vi "Create All Message Queues.vi"(8 "error in (no error)":T1 caption="entrée d'erreur (pas d'erreur)") -> (0 "error out":T1 caption="sortie d'erreur", 3 "Files d'attente de messages en sortie":T2)   [LabVIEW 2020, in "Message Queue.lvlib"]
doc: "Ce VI crée et initialise toutes les files d'attente de messages de l'application. Si votre application requiert plusieurs files d'attente de messages, cliquez sur la constante \"Message Queues\" ci-dessus avec le bouton droit et sélectionnez Ouvrir la déf. de type. Ajoutez les nouvelles files d'attente de messages à la définition de type puis initialisez-les dans ce VI."
uses:
  Message Queue.lvlib
  All Message Queues.ctl
  Message Cluster.ctl
  Enqueue Message (Single).vi
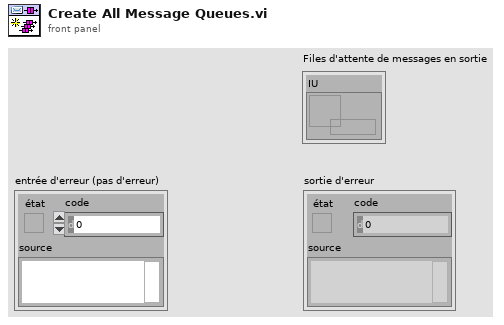
[diagram p1: front panel]
types:
  T1 = cluster{"état":bool, "code":i32, "source":string}
  T2 = typedef "Message Queue.lvlib/All Message Queues.ctl" = cluster{"IU":refnum<queue>}
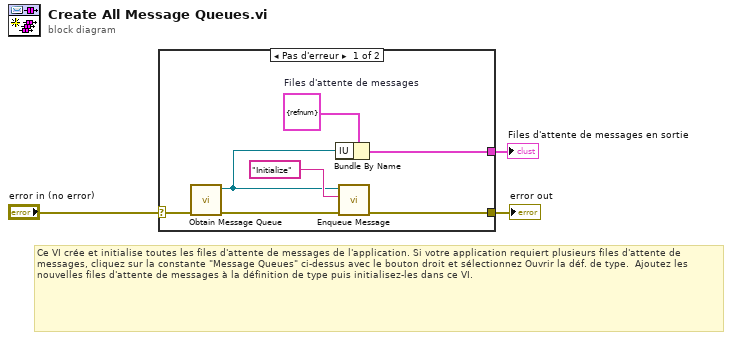
[diagram p0: block diagram]
diagram:
  # "Ce VI crée et initialise toutes les files d'attente de messages de l'application. Si votre application requiert plusieurs files d'attente de messages, cliquez sur la constante \"Message Queues\" ci-dessus avec le bouton droit et sélectionnez Ouvrir la déf. de type.  Ajoutez les nouvelles files d'attente de messages à la définition de type puis initialisez-les dans ce VI."
  n1 = case shown="Pas d'erreur" "error in (no error)" {
    selector: "error in (no error)" -> [w7 w11]
    tunnel: [w10 w11] -> w3
    tunnel: [w8 _] -> w2
    frame No Error {
      w9 = T2 {"IU"=refnum}  # Files d'attente de messages
      n2 = call "Obtain Message Queue.vi"("error in (no error)"=w7) -> ("error out"=w6:T1, "File d'attente de messages"=w4:refnum<queue>)  [unwired: 9 in]
      n3 = Bundle By Name(cluster=w9, "IU"=w4) -> (w8:T2)
      n4 = call-poly "Enqueue Message.vi"("error in (no error)"=w6, "Message"="Initialize", "File d'attente de messages"=w4) -> ("error out"=w10:T1)  [unwired: 7 in, 1 out]
    }
    frame Error {
    }
  }
  "Files d'attente de messages en sortie" <- w2
  "error out" <- w3
